vi "Get CD Refs.vi"(8 "error in (no error)":errorcluster, 11 "Device Reference in":T17 format="%.0x") -> (0 "error out":errorcluster, 2 "VS References":T1={"Properties"={"Name"="", "CAN"={"Database File"=path "", "CAN Interface"=enum."CAN1", "Baud Rate"=0, "Diagnostic Protocol"=enum."GMLAN", "Transport Protocol"=enum."ISO TP - Normal Mode", "Transmit ID"=0, "Receive ID"=0, "Transmit Extension"=2, "Receive Extension"=1, "Receive UUDT ID"=0, "Enable Stream"=TRUE, "VW TP Channel ID"=0, "Security"={"DLL Path"=path "", "Security Level"=0}}, "FPGA Settings"={"RT Bitfile Path"=path "", "RIO Device"=0, "Enable"=FALSE}, "PIDs"=[], "PID Lookup"=variant(enum16{"GMLAN", "KWP-2000", "UDS"} enum."GMLAN"), "CPIDs"=[], "CPID Lookup"=variant(u32 0), "DIDs"=[], "DID Lookup"=variant(u8 0), "DPIDs"=[], "DPID Lookup"=variant(u32 0), "DTC descriptor"={"DTC Byte Length"=2, "Status Byte Length"=1, "Add Data Byte Length"=1, "Byte Order"=enum."Motorola"}}, "Refs"={"PIDs"=[], "CPIDs"={"Refs"=[], "Values"=[]}, "DIDs"=[], "Number of DTCs"=0, "DTCs"=[], "Success"=0, "Command Chanels"=[]}} {"Refs"."Command Chanels" format="%.0x"; "Refs"."Success" format="%.0x"; "Refs"."DTCs" format="%.0x"; "Refs"."Number of DTCs" format="%.0x"; "Refs"."DIDs" format="%.0x"; "Refs"."CPIDs"."Refs"."Data Reference" format="%.0x"; "Refs"."PIDs" format="%.0x"; "Properties"."CPIDs"."Signals"."Byte Order" items=["Little Endian", "Big Endian"]; "Properties"."CPIDs"."Signals"."Data Type" items=["Signed", "Unsigned", "IEEE Float"]; "Properties"."DIDs"."Signals"."Byte Order" items=["Little Endian", "Big Endian"]; "Properties"."DIDs"."Signals"."Data Type" items=["Signed", "Unsigned", "IEEE Float"]; "Properties"."CAN"."VW TP Channel ID" format="%.0x"; "Properties"."CAN"."Receive UUDT ID" format="%.0x"; "Properties"."CAN"."Receive Extension" format="%.0x"; "Properties"."CAN"."Transmit Extension" format="%.0x"; "Properties"."CAN"."Receive ID" format="%.0x"; "Properties"."CAN"."Transmit ID" format="%.0x"; "Properties"."PIDs"."Signals"."Byte Order" items=["Little Endian", "Big Endian"]; "Properties"."PIDs"."Signals"."Data Type" items=["Signed", "Unsigned", "IEEE Float"]}, 3 "Device Reference out":T17 format="%.0x")   [LabVIEW 2015, in "Diagnostics Addon Engine.lvlib"]
uses:
  Diagnostics Addon Engine.lvlib
  <vilib>/NI Veristand/Custom Device API/Custom Device Item Ref.ctl
  Compiled.Settings
  Section Properties.ctl
  Shared/CAN Configuration.ctl
  Shared/CAN Interface.ctl
  Shared/Diagnostic Protocols.ctl
  Shared/Transport Protocols.ctl
  Shared/Security.ctl
  Shared/FPGA Bitfile Settings.ctl
  Shared/DIDPID Parameters.ctl
  Shared/DIDPID Signal Parameters.ctl
  Shared/DPID Parameters.ctl
  Shared/DPID Periodic Rate.ctl
  <vilib>/Automotive Diagnostic Command Set/Diagnostic Protocols.llb/DTC Descriptor.ctl
  Shared/Compiled.Refs.ctl
  <vilib>/NI Veristand/Custom Device API/Data Reference.ctl
  <vilib>/NI Veristand/Custom Device API/Block Data Reference.ctl
  <vilib>/NI Veristand/Custom Device API/Data Access Type.ctl
  Shared/FG Action.ctl
  Shared/ID FG.vi
  Shared/Get DIDPID.vi
  Shared/Calculate DIDPID Frame Length.vi
  Shared/Get Signals from DIDPID.vi
  Shared/Signal Parameters FG.vi
  <vilib>/NI Veristand/Custom Device API/NI VeriStand - Get Item Property.vi
  <vilib>/NI Veristand/Custom Device API/Get Item Property (Variant).vi
  <vilib>/NI Veristand/Custom Device API/NI VeriStand - Set Item Property.vi
  <vilib>/NI Veristand/Custom Device API/Set Item Property (Variant).vi
  Shared/GUID Lookup.vi
  <vilib>/NI Veristand/Custom Device Tools/Custom Device Utility Library/NI VeriStand - Search for Item by GUID.vi
  <vilib>/NI Veristand/Custom Device API/Set Item Property (U32).vi
  <vilib>/NI Veristand/Custom Device API/Set Item Property (Path).vi
  <vilib>/NI Veristand/Custom Device API/Set Item Property (Boolean).vi
  <vilib>/NI Veristand/Custom Device API/Get Item Property (U32).vi
  <vilib>/NI Veristand/Custom Device API/Get Item Property (Path).vi
  <vilib>/NI Veristand/Custom Device API/Get Item Property (Boolean).vi
  <vilib>/NI Veristand/Custom Device Tools/Custom Device Utility Library/NI VeriStand - Search for Item by Name.vi
  <vilib>/NI Veristand/Custom Device API/NI VeriStand - Get Custom Device Channel Data.vi
  <vilib>/NI Veristand/Custom Device API/NI VeriStand - Get Item Description.vi
  <vilib>/NI Veristand/Custom Device API/Get Item Property (String).vi
  <vilib>/NI Veristand/Custom Device API/Get Item Property (Double).vi
  <vilib>/NI Veristand/Custom Device API/Set Item Property (String).vi
  <vilib>/NI Veristand/Custom Device API/Set Item Property (Double).vi
  <vilib>/NI Veristand/Custom Device API/NI VeriStand - Get Channel Block Data References.vi
  <vilib>/NI Veristand/Custom Device Tools/Custom Device Utility Library/Custom Device Utility Library.lvlib
  Shared/Diagnostics Addon Shared.lvlib
  <vilib>/NI Veristand/Custom Device API/Custom Device API.lvlib
  System Explorer/Diagnostics Addon System Explorer.lvlib
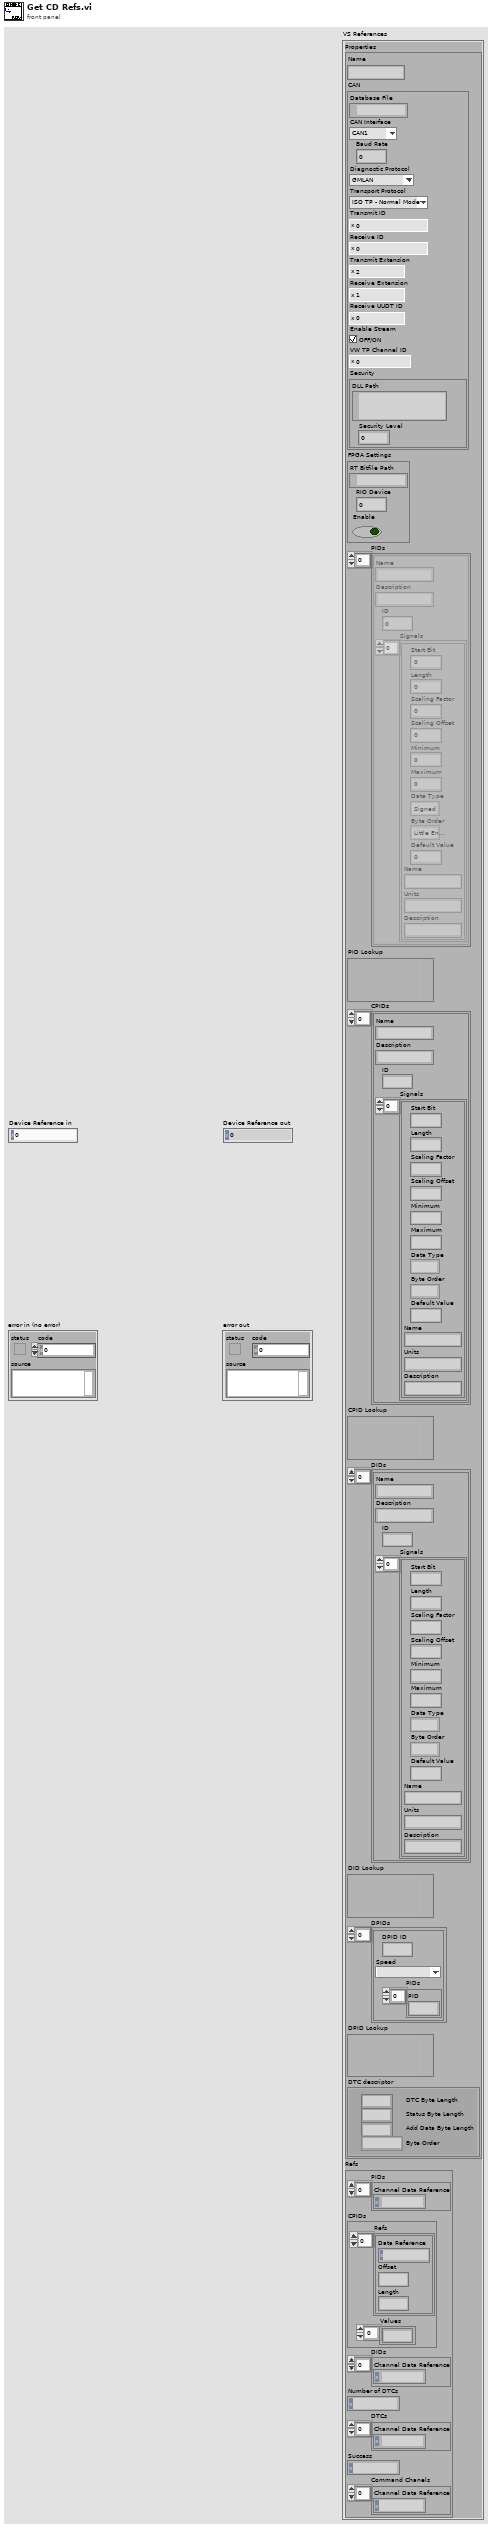
[diagram p1: front panel]
types:
  T1 = typedef "Diagnostics Addon Engine.lvlib/Compiled.Settings" = cluster{"Properties":T2, "Refs":T14}
  T2 = typedef "Diagnostics Addon Engine.lvlib/Section Properties.ctl" = cluster{"Name":string, "CAN":T3, "FPGA Settings":T8, "PIDs":T9[], "PID Lookup":variant, "CPIDs":T9[], "CPID Lookup":variant, "DIDs":T9[], "DID Lookup":variant, "DPIDs":T11[], "DPID Lookup":variant, "DTC descriptor":T13}
  T3 = typedef "Diagnostics Addon Shared.lvlib/CAN Configuration.ctl" = cluster{"Database File":path, "CAN Interface":T4, "Baud Rate":u32, "Diagnostic Protocol":T5, "Transport Protocol":T6, "Transmit ID":u32, "Receive ID":u32, "Transmit Extension":u8, "Receive Extension":u8, "Receive UUDT ID":u32, "Enable Stream":bool, "VW TP Channel ID":u32, "Security":T7}
  T4 = typedef "Diagnostics Addon Shared.lvlib/CAN Interface.ctl" = enum16{"CAN0", "CAN1", "CAN2", "CAN3", "CAN4", "CAN5", "CAN6", "CAN7", "CAN8", "CAN9", "CAN10", "CAN11", "CAN12", "CAN13", "CAN14", "CAN15", "CAN16", "CAN17", "CAN18", "CAN19", "CAN20", "CAN21", "CAN22", "CAN23", "CAN24", "CAN25", "CAN26", "CAN27", "CAN28", "CAN29", "CAN30", "CAN31", "CAN32", "CAN33", "CAN34", "CAN35", "CAN36", "CAN37", "CAN38", "CAN39", "CAN40", "CAN41", "CAN42", "CAN43", "CAN44", "CAN45", "CAN46", "CAN47", "CAN48", "CAN49", "CAN50", "CAN51", "CAN52", "CAN53", "CAN54", "CAN55", "CAN56", "CAN57", "CAN58", "CAN59", "CAN60", "CAN61", "CAN62", "CAN63", "CAN 256 (Virtual)", "CAN 257 (Virtual)"}
  T5 = typedef "Diagnostics Addon Shared.lvlib/Diagnostic Protocols.ctl" = enum16{"GMLAN", "KWP-2000", "UDS"}
  T6 = typedef "Diagnostics Addon Shared.lvlib/Transport Protocols.ctl" = enum16{"ISO TP - Normal Mode", "ISO TP - Mixed Mode", "VW TP 2.0", "Diagnostics on IP"}
  T7 = typedef "Diagnostics Addon Shared.lvlib/Security.ctl" = cluster{"DLL Path":path, "Security Level":u8}
  T8 = typedef "Diagnostics Addon Shared.lvlib/FPGA Bitfile Settings.ctl" = cluster{"RT Bitfile Path":path, "RIO Device":u16, "Enable":bool}
  T9 = typedef "Diagnostics Addon Shared.lvlib/DIDPID Parameters.ctl" = cluster{"Name":string, "Description":string, "ID":u16, "Signals":T10[]}
  T10 = typedef "Diagnostics Addon Shared.lvlib/DIDPID Signal Parameters.ctl" = cluster{"Start Bit":u8, "Length":u8, "Scaling Factor":dbl, "Scaling Offset":dbl, "Minimum":dbl, "Maximum":dbl, "Data Type":u32, "Byte Order":u32, "Default Value":dbl, "Name":string, "Units":string, "Description":string}
  T11 = typedef "Diagnostics Addon Shared.lvlib/DPID Parameters.ctl" = cluster{"DPID ID":u8, "Speed":T12, "PIDs":u16[]}
  T12 = typedef "Diagnostics Addon Shared.lvlib/DPID Periodic Rate.ctl" = enum16{"Slow", "Medium", "Fast"}
  T13 = typedef "DTC Descriptor.ctl" = cluster{"DTC Byte Length":i32, "Status Byte Length":i32, "Add Data Byte Length":i32, "Byte Order":enum16{"Motorola", "Intel"}}
  T14 = typedef "Diagnostics Addon Shared.lvlib/Compiled.Refs.ctl" = cluster{"PIDs":T15[], "CPIDs":cluster{"Refs":T16[], "Values":dbl[]}, "DIDs":T15[], "Number of DTCs":T15, "DTCs":T15[], "Success":T15, "Command Chanels":T15[]}
  T15 = typedef "Custom Device API.lvlib/Data Reference.ctl" = i32
  T16 = typedef "Custom Device API.lvlib/Block Data Reference.ctl" = cluster{"Data Reference":T15, "Offset":u64, "Length":u64}
  T17 = typedef "Custom Device API.lvlib/Custom Device Item Ref.ctl" = u64
  T18 = typedef "Diagnostics Addon Shared.lvlib/FG Action.ctl" = enum16{"Get", "Set"}
  T19 = typedef "Custom Device API.lvlib/Data Access Type.ctl" = enum16{"Read", "Write"}
  T20 = typedef "Diagnostics Addon Engine.lvlib/DIDPID Signal VS References.ctl" = cluster{"ID":u16, "Signal Refs":T17[]}
  T21 = typedef "Custom Device API.lvlib/Custom Device Item Info.ctl" = cluster{"Name":string, "Is Channel":bool, "GUID":string, "Is Waveform":bool}
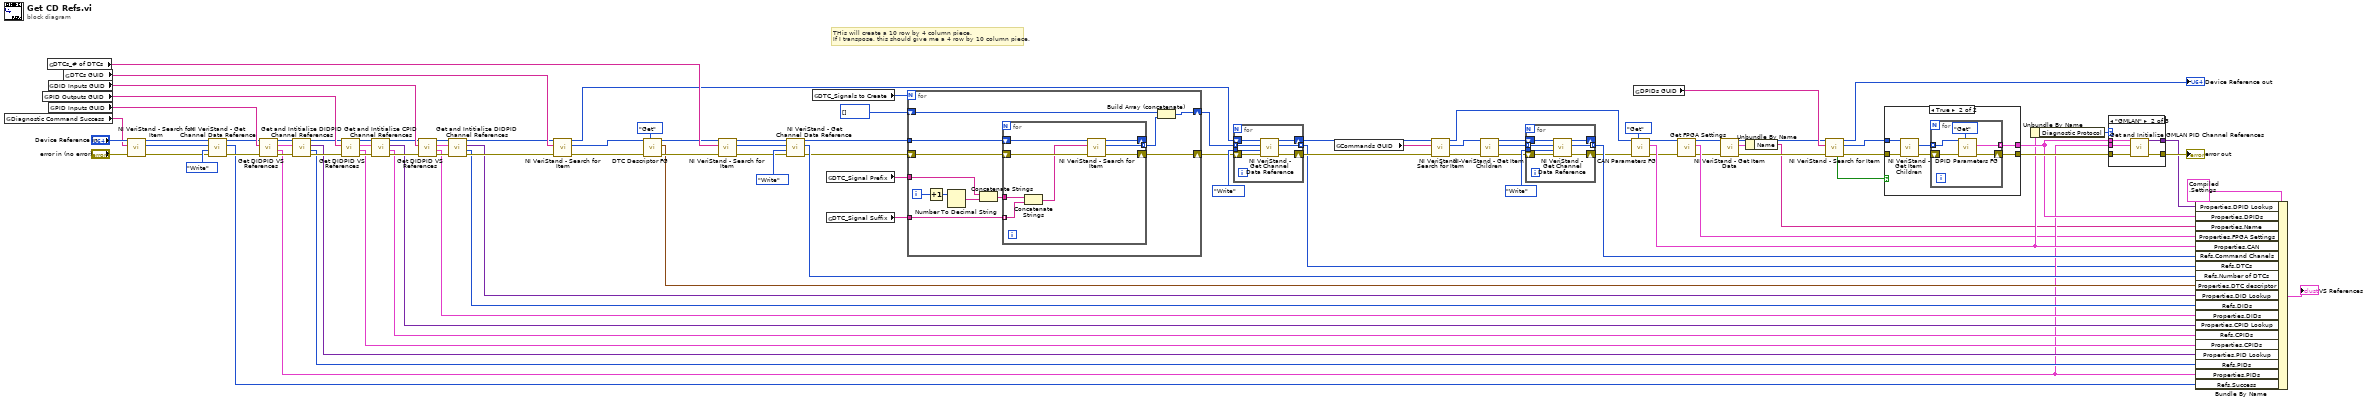
[diagram p0: block diagram]
diagram:
  # "THis will create a 10 row by 4 column piece.\nIf I transpose, this should give me a 4 row by 10 column piece."
  n1 = global read "GUID Lookup.vi" "Diagnostic Command Success"() -> (w89:string)
  n2 = global read "GUID Lookup.vi" "PID Outputs GUID"() -> (w83:string)
  n3 = global read "GUID Lookup.vi" "DTCs_# of DTCs"() -> (w95:string)
  n4 = global read "GUID Lookup.vi" "DID Inputs GUID"() -> (w84:string)
  n5 = global read "GUID Lookup.vi" "PID Inputs GUID"() -> (w82:string)
  n6 = global read "GUID Lookup.vi" "DTCs GUID"() -> (w96:string)
  n7 = call-poly <vilib>:"NI VeriStand - Search for Item.vi"("error in"="error in (no error)", "Item Name"=w89, "Section Ref in"="Device Reference in") -> ("error out"=w47:errorcluster, "Item Ref"=w43:T17, "Section Ref out"=w45:T17)  [unwired: 5 in, 1 out]
  n8 = call <vilib>:"NI VeriStand - Get Channel Data Reference.vi"("error in (no error)"=w47, "Access"=Data_Access_Type."Write", "Channel Ref in"=w43, "Device Ref in"=w45) -> ("error out"=w46:errorcluster, "Channel Data Reference"=w42:T15, "Device Ref out"=w44:T17)  [unwired: 5 in]
  n9 = call "Get DIDPID VS References.vi"("error in (no error)"=w46, "GUID"=w82, "Section Ref in"=w44) -> ("error out"=w74:errorcluster, "Frame Settings Array"=w14:T9[], "Frame Refs"=w72:T20[], "Section Ref out"=w76:T17)  [unwired: 5 in]
  n10 = call "Get and Intitialize DIDPID Channel References.vi"("error in (no error)"=w74, "Refs"=w72, "Item Ref in"=w76) -> ("error out"=w73:errorcluster, "Refs"=w41:T15[], "Lookup Table"=w22:variant, "Item Ref out"=w75:T17)  [unwired: 5 in]
  n11 = call "Get DIDPID VS References.vi"("error in (no error)"=w73, "GUID"=w83, "Section Ref in"=w75) -> ("error out"=w66:errorcluster, "Frame Settings Array"=w21:T9[], "Frame Refs"=w62:T20[], "Section Ref out"=w64:T17)  [unwired: 5 in]
  n12 = call "Get and Intitialize CPID Channel References.vi"("error in (no error)"=w66, "Refs"=w62, "Item Ref in"=w64) -> ("error out"=w65:errorcluster, "output cluster"=w40:cluster{"Refs":T16[], "Values":dbl[]}, "Lookup Table"=w20:variant, "Item Ref out"=w63:T17)  [unwired: 5 in]
  n13 = call "Get DIDPID VS References.vi"("error in (no error)"=w65, "GUID"=w84, "Section Ref in"=w63) -> ("error out"=w70:errorcluster, "Frame Settings Array"=w19:T9[], "Frame Refs"=w71:T20[], "Section Ref out"=w68:T17)  [unwired: 5 in]
  n14 = call "Get and Intitialize DIDPID Channel References.vi"("error in (no error)"=w70, "Refs"=w71, "Item Ref in"=w68) -> ("error out"=w69:errorcluster, "Refs"=w39:T15[], "Lookup Table"=w18:variant, "Item Ref out"=w67:T17)  [unwired: 5 in]
  n15 = call-poly <vilib>:"NI VeriStand - Search for Item.vi"("error in"=w69, "Item GUID"=w96, "Section Ref in"=w67) -> ("error out"=w28:errorcluster, "Item Ref"=w26:T17, "Section Ref out"=w57:T17)  [unwired: 5 in, 1 out]
  n16 = call "DTC Descriptor FG.vi"("Action"=FG_Action."Get", "error in (no error)"=w28, "Device Item Ref in"=w26) -> ("error out"=w27:errorcluster, "DTC descriptor"=w17:T13, "Device Item Ref out"=w25:T17)  [unwired: 6 in]
  n17 = call-poly <vilib>:"NI VeriStand - Search for Item.vi"("error in"=w27, "Item Name"=w95, "Section Ref in"=w25) -> ("error out"=w52:errorcluster, "Item Ref"=w55:T17, "Section Ref out"=w50:T17)  [unwired: 5 in, 1 out]
  n18 = call <vilib>:"NI VeriStand - Get Channel Data Reference.vi"("error in (no error)"=w52, "Access"=Data_Access_Type."Write", "Channel Ref in"=w55, "Device Ref in"=w50) -> ("error out"=w51:errorcluster, "Channel Data Reference"=w54:T15, "Device Ref out"=w49:T17)  [unwired: 5 in]
  n19 = global read "GUID Lookup.vi" "DTC_Signals to Create"() -> (w92:i32)
  n20 = global read "GUID Lookup.vi" "DTC_Signal Prefix"() -> (w94:string)
  n21 = global read "GUID Lookup.vi" "DTC_Signal Suffix"() -> (w93:string[])
  n22 = for {
    N: w92 -> [_]
    tunnel: w49 -> [w108]
    shift-right: [w106] -> w60
    shift-left: w51 -> [w107]
    tunnel: w93 -> [w101]
    tunnel: w94 -> [w100]
    shift-right: [w97] -> w58
    shift-left: T17[] [] -> [w99]
    i -> [w103]
    n23 = Increment(x=w103) -> (x+1=w105:i32)
    n24 = Number To Decimal String(number=w105) -> (decimal integer string=w104:string)  [unwired: 1 in]
    n25 = Concatenate Strings(w100, w104) -> (w102:string)
    n26 = for {
      shift-right: [w115] -> _
      shift-left: w108 -> [w116]
      shift-right: [w113] -> w106
      shift-left: w107 -> [w114]
      tunnel: w101 -> [w112] mode=indexing
      tunnel: w102 -> [w111]
      tunnel: [w109] -> w98 mode=indexing
      n27 = Concatenate Strings(w111, w112) -> (w110:string)
      n28 = call-poly <vilib>:"NI VeriStand - Search for Item.vi"("error in"=w114, "Item Name"=w110, "Section Ref in"=w116) -> ("error out"=w113:errorcluster, "Item Ref"=w109:T17, "Section Ref out"=w115:T17)  [unwired: 5 in, 1 out]
    }
    n29 = Build Array (concatenate)(w99, w98) -> (w97:T17[])
  }
  n30 = for {
    tunnel: w58 -> [w119] mode=indexing
    tunnel: Data_Access_Type."Write" ("Access") -> [w118]
    shift-right: [w121] -> w59
    shift-left: w60 -> [w122]
    shift-right: [w123] -> w56
    shift-left: w57 -> [w120]
    tunnel: [w117] -> w9 mode=indexing
    n31 = call <vilib>:"NI VeriStand - Get Channel Data Reference.vi"("error in (no error)"=w122, "Access"=w118, "Channel Ref in"=w119, "Device Ref in"=w120) -> ("error out"=w121:errorcluster, "Channel Data Reference"=w117:T15, "Device Ref out"=w123:T17)  [unwired: 5 in]
  }
  n32 = global read "GUID Lookup.vi" "Commands GUID"() -> (w87:string)
  n33 = call-poly <vilib>:"NI VeriStand - Search for Item.vi"("error in"=w59, "Item GUID"=w87, "Section Ref in"=w56) -> ("error out"=w86:errorcluster, "Item Ref"=w85:T17, "Section Ref out"=w30:T17)  [unwired: 5 in, 1 out]
  n34 = call <vilib>:"NI VeriStand - Get Item Children.vi"("error in (no error)"=w86, "Item Ref in"=w85) -> ("error out"=w80:errorcluster, "Child Refs"=w78:T17[], "Item Ref out"=w79:T17)  [unwired: 6 in, 1 out]
  n35 = for {
    tunnel: w78 -> [w126] mode=indexing
    tunnel: Data_Access_Type."Write" ("Access") -> [w125]
    shift-right: [w128] -> w32
    shift-left: w80 -> [w129]
    shift-right: [w130] -> _
    shift-left: w79 -> [w127]
    tunnel: [w124] -> w77 mode=indexing
    n36 = call <vilib>:"NI VeriStand - Get Channel Data Reference.vi"("error in (no error)"=w129, "Access"=w125, "Channel Ref in"=w126, "Device Ref in"=w127) -> ("error out"=w128:errorcluster, "Channel Data Reference"=w124:T15, "Device Ref out"=w130:T17)  [unwired: 5 in]
  }
  n37 = call "CAN Parameters FG.vi"("Action"=FG_Action."Get", "error in (no error)"=w32, "Device Item Ref in"=w30) -> ("error out"=w12:errorcluster, "Diagnostics Basic Configuraiton"=w15:T3, "Device Item Ref out"=w11:T17)  [unwired: 6 in]
  n38 = global read "GUID Lookup.vi" "DPIDs GUID"() -> (w37:string)
  n39 = call "Get FPGA Settings.vi"("error in (no error)"=w12, "Item Ref in"=w11) -> ("error out"=w5:errorcluster, "FPGA Bitfile Settings"=w10:T8, "Item Ref out"=w3:T17)  [unwired: 7 in]
  n40 = call <vilib>:"NI VeriStand - Get Item Data.vi"("error in (no error)"=w5, "Item Ref in"=w3) -> ("error out"=w4:errorcluster, "Item Info"=w6:T21, "Item Ref out"=w2:T17)  [unwired: 6 in, 1 out]
  n41 = Unbundle By Name(w6) -> ("Name"=w1:string)
  n42 = call-poly <vilib>:"NI VeriStand - Search for Item.vi"("error in"=w4, "Item GUID"=w37, "Section Ref in"=w2) -> ("error out"=w38:errorcluster, "Item Ref"=w36:T17, "Section Ref out"=→"Device Reference out":T17, "Found"=w34:bool)  [unwired: 5 in]
  n43 = case shown="True" w34 {
    tunnel: w38 -> [w131 w137]
    tunnel: w36 -> [_ w134]
    tunnel: [w131 w133] -> w24
    tunnel: [_ w132] -> w16
    frame False {
    }
    frame True {
      n44 = call <vilib>:"NI VeriStand - Get Item Children.vi"("error in (no error)"=w137, "Item Ref in"=w134) -> ("error out"=w136:errorcluster, "Child Refs"=w135:T17[])  [unwired: 6 in, 2 out]
      n45 = for {
        tunnel: w135 -> [w141] mode=indexing
        tunnel: [w140] -> w132 mode=indexing
        shift-right: [w139] -> w133
        shift-left: w136 -> [w142]
        n46 = call "DPID Parameters FG.vi"("Action"=FG_Action."Get", "error in (no error)"=w142, "Device Item Ref in"=w141) -> ("error out"=w139:errorcluster, "DPID"=w140:T11)  [unwired: 6 in, 1 out]
      }
    }
  }
  n47 = Unbundle By Name(w15) -> ("Diagnostic Protocol"=w33:T5)
  n48 = case shown="\"GMLAN\"" w33 {
    tunnel: w14 -> [_ w145 _]
    tunnel: [w143 w148 w149] -> w31
    tunnel: w24 -> [w143 w147 w149]
    tunnel: [_ w146 _] -> w13
    tunnel: w16 -> [_ w144 _]
    frame "KWP-2000" {
    }
    frame "GMLAN" {
      n49 = call "Get and Initialize GMLAN PID Channel References.vi"("error in (no error)"=w147, "PIDs"=w145, "DPIDs"=w144) -> ("error out"=w148:errorcluster, "Lookup Table"=w146:variant)  [unwired: 7 in]
    }
    frame "UDS" {
    }
  }
  "error out" <- w31
  n50 = Bundle By Name(cluster=T1 {"Properties"={"Name"="", "CAN"={"Database File"=path "", "CAN Interface"=enum."CAN1", "Baud Rate"=0, "Diagnostic Protocol"=enum."GMLAN", "Transport Protocol"=enum."ISO TP - Normal Mode", "Transmit ID"=0, "Receive ID"=0, "Transmit Extension"=2, "Receive Extension"=1, "Receive UUDT ID"=0, "Enable Stream"=TRUE, "VW TP Channel ID"=0, "Security"={"DLL Path"=path "", "Security Level"=0}}, "FPGA Settings"={"RT Bitfile Path"=path "", "RIO Device"=0, "Enable"=FALSE}, "PIDs"=[], "PID Lookup"=variant(enum16{"GMLAN", "KWP-2000", "UDS"} enum."GMLAN"), "CPIDs"=[], "CPID Lookup"=variant(u32 0), "DIDs"=[], "DID Lookup"=variant(u8 0), "DPIDs"=[], "DPID Lookup"=variant(u32 0), "DTC descriptor"={"DTC Byte Length"=2, "Status Byte Length"=1, "Add Data Byte Length"=1, "Byte Order"=enum."Motorola"}}, "Refs"={"PIDs"=[], "CPIDs"={"Refs"=[], "Values"=[]}, "DIDs"=[], "Number of DTCs"=0, "DTCs"=[], "Success"=0, "Command Chanels"=[]}} ("VS References"), "Properties.DPID Lookup"=w13, "Properties.DPIDs"=w16, "Properties.Name"=w1, "Properties.FPGA Settings"=w10, "Properties.CAN"=w15, "Refs.Command Chanels"=w77, "Refs.DTCs"=w9, "Refs.Number of DTCs"=w54, "Properties.DTC descriptor"=w17, "Properties.DID Lookup"=w18, "Refs.DIDs"=w39, "Properties.DIDs"=w19, "Properties.CPID Lookup"=w20, "Refs.CPIDs"=w40, "Properties.CPIDs"=w21, "Properties.PID Lookup"=w22, "Refs.PIDs"=w41, "Properties.PIDs"=w14, "Refs.Success"=w42) -> (→"VS References":T1)
